vi "FPGATest.vi"() -> ()   [LabVIEW 2016]
uses:
  <vilib>/Platform/TimedLoop/XDataNode/timing_clust.ctl
  <vilib>/Platform/TimedLoop/XDataNode/nitl_modes.ctl
  <vilib>/Platform/TimedLoop/XDataNode/wakeup.ctl
  <userlib>/_NI SPI IP/FPGA/Controllers/Public/Transfer Settings.ctl
  <vilib>/rvi/Emulation/niFpgaGetClockAttributes.vi
  <vilib>/rvi/Emulation/niFpgaSctlEmulationGetInTimedLoop.vi
  <vilib>/rvi/Emulation/niFpgaEmulationReportErrorSimple.vi
  <vilib>/rvi/DataTransferAndStorage/Container/Common/niFpgaContainerGetUniqueNameForEmu.vi
  <vilib>/rvi/DataTransferAndStorage/Container/Common/niFpgaContainerSetEmuInfo.vi
  <vilib>/rvi/eio/common/nirviEmuReportErrorAndStop.vi
  <vilib>/rvi/DataTransferAndStorage/Container/Common/niFpgaContainerExecOnDevCompGetState.vi
  <vilib>/rvi/Emulation/niFpgaEmulationIsFPGAContextNoSignature.vi
  <vilib>/rvi/Memory/Memory_Emulation/niFpgaMemoryEmulationCacheClearOnFirstRun.vi
  <vilib>/rvi/Memory/Memory_Emulation/nirvimemoryEmulationManagerCache_MakeExclusive.vi
  <vilib>/rvi/Memory/Memory_Emulation/niFpgaMemoryEmulationValidateCache.vi
  <vilib>/rvi/Memory/Memory_Emulation/nirvimemoryEmulationManagerCache_InsertValue.vi
  <vilib>/Utility/error.llb/Clear Errors.vi
  <vilib>/rvi/Memory/Memory_Emulation/nirvimemoryEmulationManagerCache_ReleaseExclusive.vi
  <vilib>/rvi/Memory/Memory_Emulation/nirvimemoryEmulationManagerCache_GetValue.vi
  <vilib>/rvi/Memory/Memory_Emulation/nirvimemoryEmulationManagerCache_SetValue.vi
  <vilib>/rvi/Emulation/niFpgaProcessEmulError.vi
  <vilib>/rvi/Emulation/niFpgaCriticalErrorInLSC.vi
  <vilib>/rvi/eio/common/nirviEmuTemplateMethod_errors.vi
  <vilib>/Platform/TimedLoop/XDataNode/XDataNode.xnode
  <vilib>/rvi/LocalResourceManager/LocalResourceManager.xnode
  <vilib>/rvi/DataTransferAndStorage/Container/XNode/niFpgaContainer.xnode
  <vilib>/rvi/DataTransferAndStorage/Register/Emulation/niFpgaRegisterEmulationRefIn.vi
  <vilib>/eio/EIONode/EIONode.xnode
  <userlib>/_NI SPI IP/FPGA/Controllers/NI SPI IP FPGA.lvlib
  <vilib>/Platform/TimedLoop/XDataNode/XDNodeRunTimeDep.lvlib
panel:
  in  "CS":bool=TRUE
  in  "CE":bool=TRUE
  out "ByteOut":u8
  in  "ByteIn":u8 format="%x"
  in  "NewData":bool=TRUE
  in  "Mode":enum16{"ReadWrite", "Raw"}(ring)
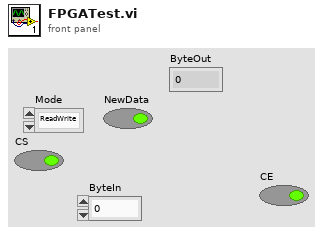
[diagram p1: front panel]
types:
  T1 = typedef "XDNodeRunTimeDep.lvlib/timing_clust.ctl" = cluster{"Expected End [f-1]":u64, "Actual End [f-1]":u64, "Finished Late? [f-1]":bool, "Expected End [i-1]":u64, "Actual End [i-1]":u64, "Finished Late? [i-1]":bool, "Expected Start [i]":u64, "Actual Start [i]":u64, "Expected Start [f]":u64, "Actual Start [f]":u64, "Source Name":string, "Structure Name":string, "Period":i64, "Deadline":i64, "Offset":i64, "Start":i64, "Priority":i32, "Timeout":i32, "Mode":T2, "Wakeup Reason":T3, "Error":errorcluster, "Source Type":string, "Secondary Source Type":string, "Global End Time":u64, "Global Start Time":u64, "Frame Duration":u64, "Iteration Duration":u64, "Assigned CPU":i32, "I/O Scan Engine Mode":u32}
  T2 = typedef "XDNodeRunTimeDep.lvlib/nitl_modes.ctl" = enum32{"No Change", "Process missed periods, maintain original phase", "Discard missed periods, maintain original phase", "Process missed periods, ignore original phase", "Discard missed periods, ignore original phase"}
  T3 = typedef "XDNodeRunTimeDep.lvlib/wakeup.ctl" = enum32{"Normal", "Aborted", "Asynchronous wakeup", "Timing source error", "Timed loop error", "Timeout"}
  T4 = typedef "NI SPI IP FPGA.lvlib/Transfer Settings.ctl" = cluster{"Divide Value":u8, "Transfer Length (bits)":u8, "CS Asserted Polarity":bool, "Clock Polarity (CPOL)":bool, "Clock Phase (CPHA)":bool, "Lengthen MISO Setup":bool, "Direction Change Bit":u8, "MOSI Starts as Output":bool, "Tristatable MOSI":bool}
  T5 = typedef "NI SPI IP FPGA.lvlib/Spi Master Outputs.ctl" = cluster{"Chip Select":bool, "Clock":bool, "MOSI":bool, "MOSI OE":bool}
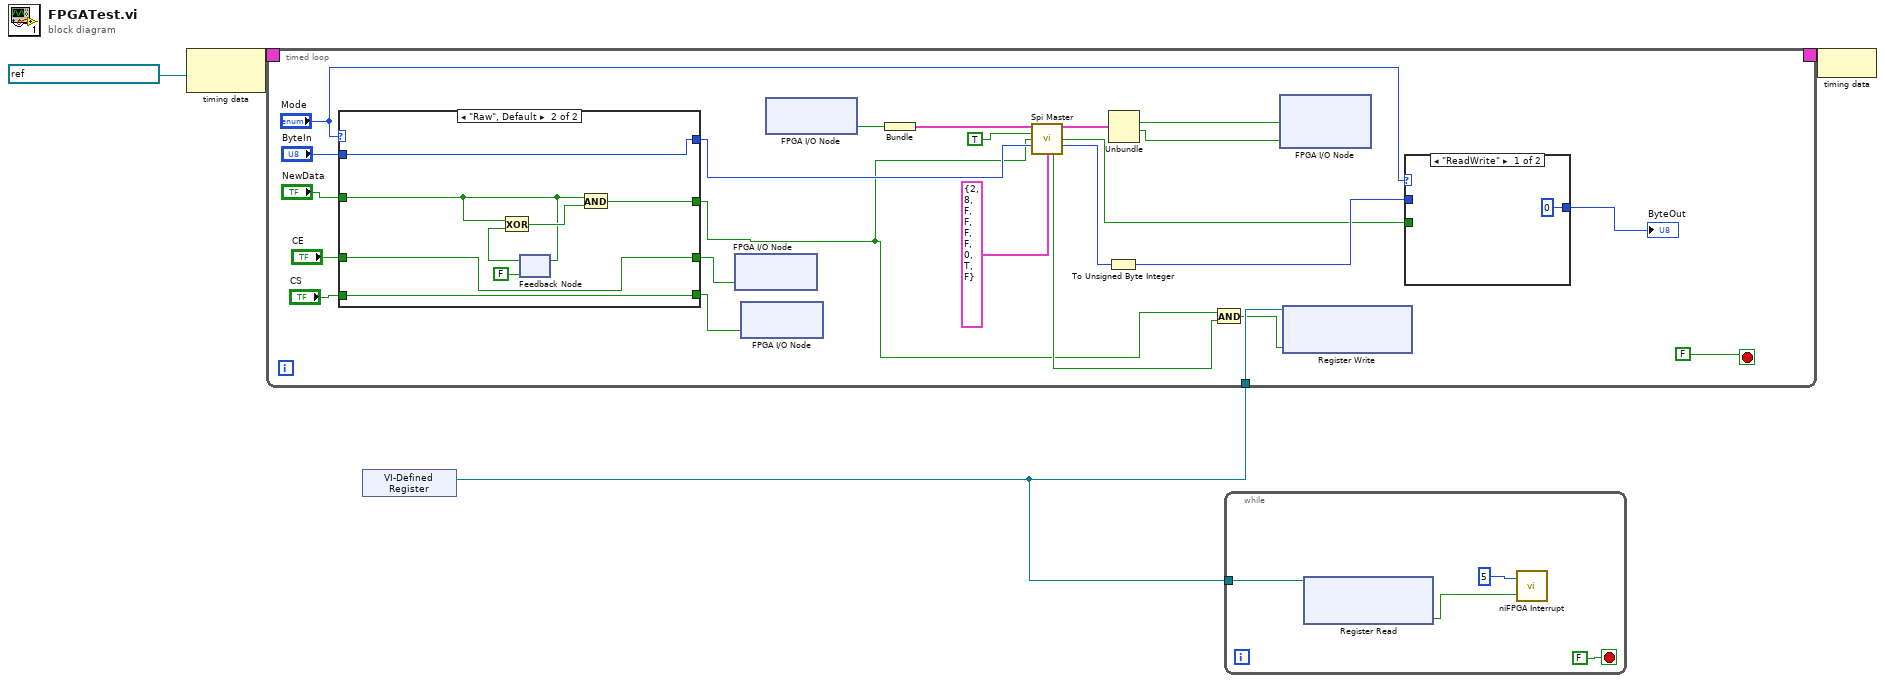
[diagram p0: block diagram]
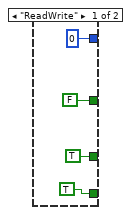
[diagram p3: hidden frame]
diagram:
  n1 = node-c288(refnum<k21> "40 MHz Onboard Clock" ("Source Name")) -> (w4:T1)
  n2 = xnode "VI-Defined Register"() -> ("Register Out"=w2:refnum<k21>)
  n3 = timed-loop {
    timing: w4 -> [_]
    timing-out: [_] -> w3
    tunnel: w2 -> [w12]
    stop <- FALSE stop-if-true
    n4 = case shown="\"Raw\", Default" "Mode" {
      tunnel: [u8 0 ("ByteIn") w36] -> w18
      tunnel: [FALSE w39] -> w17
      tunnel: [TRUE w38] -> w19
      tunnel: "CE" -> [_ w38]
      tunnel: "NewData" -> [_ w37]
      tunnel: "ByteIn" -> [_ w36]
      tunnel: [TRUE w35] -> w6
      tunnel: "CS" -> [_ w35]
      frame "ReadWrite" {
      }
      frame "Raw", Default {
        n5 = feedback-in #1(w37) -> ()
        n6 = feedback #1(FALSE) -> (w42:bool)
        n7 = Exclusive Or(1:w42, 2:w37) -> (0:w40:bool)
        n8 = And(x=w37, y=w40) -> (x .and. y?=w39:bool)
      }
    }
    n9 = xnode "FPGA I/O Node"("SPI CS1"=w19) -> ()  [unwired: 1 in, 1 out]
    n10 = xnode "FPGA I/O Node"("SPI CS0"=w6) -> ()  [unwired: 1 in, 1 out]
    n11 = xnode "FPGA I/O Node"() -> ("SPI MISO"=w23:bool)  [unwired: 1 in, 1 out]
    n12 = Bundle("SPI MISO"=w23) -> (w25:cluster{"SPI MISO":bool})  [unwired: 1 in]
    n13 = call <userlib>:"Spi Master.vi"("spi input"=w25, "manual assert chip select"=TRUE, "start strobe"=w17, "data to write"=w18, "spi transfer settings"=T4 {"Divide Value"=2, "Transfer Length (bits)"=8, "CS Asserted Polarity"=FALSE, "Clock Polarity (CPOL)"=FALSE, "Clock Phase (CPHA)"=FALSE, "Lengthen MISO Setup"=FALSE, "Direction Change Bit"=0, "MOSI Starts as Output"=TRUE, "Tristatable MOSI"=FALSE}) -> ("spi output"=w22:T5, "read data valid"=w14:bool, "read data"=w28:u64, "ready for input"=w20:bool)  [unwired: 7 in]
    n14 = To Unsigned Byte Integer(number=w28) -> (unsigned 8bit integer=w15:u8)
    n15 = Unbundle(w22) -> ("Clock"=w21:bool, "MOSI"=w24:bool)  [unwired: 2 out]
    n16 = And(x=w17, y=w20) -> (x .and. y?=w11:bool)
    n17 = xnode "FPGA I/O Node"("SPI CLK"=w21, "SPI MOSI"=w24) -> ()  [unwired: 2 in, 2 out]
    n18 = xnode ("Register Write")("Data"=w11, "Register In"=w12) -> ()  [unwired: 1 out]
    n19 = case shown="\"ReadWrite\"" "Mode" {
      tunnel: w15 -> [_ w30]
      tunnel: w14 -> [_ _]
      tunnel: [u8 0 w30] -> w5
      frame "ReadWrite" {
      }
      frame "Raw", Default {
      }
    }
    "ByteOut" <- w5
  }
  n20 = while {
    tunnel: w2 -> [w46]
    stop <- FALSE stop-if-true
    n21 = xnode ("Register Read")("Register In"=w46) -> ("Data"=w45:bool)  [unwired: 1 out]
    n22 = call <vilib>:"niFPGA Interrupt.vi"("Wait Until Cleared (F)"=w45, "IRQ Number (0)"=u8 5) -> ()  [unwired: 1 in]
  }
  n23 = node-c288(w3) -> ()
